vi "variables_globales.vi"() -> ()   [LabVIEW 2017]
panel:
  out "Son":waveform(dbl)[](graph)
  out "stop":bool
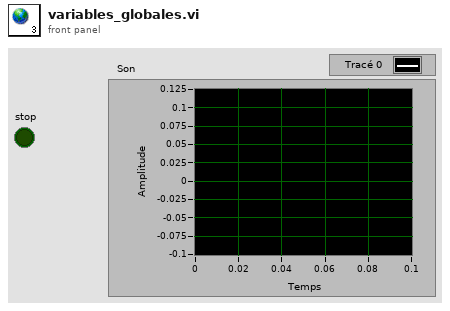
[diagram p1: front panel]
diagram:
